vi "Calibrations.vi"() -> ()   [LabVIEW 2014]
panel:
  in  "Calibrations File Location":path=path "C:/ni-rt/startup/Calibrations.txt"
  in  "Gyro gain":dbl=0.007
  in  "Rear Right Encoder Correction Factor":dbl=1.17
  in  "Rear Left Encoder Correction Factor":dbl=5.99
  in  "Front Left Encoder Correction Factor":dbl=5.09
  in  "Front Right Encoder Correction Factor":dbl=1.3
  in  "Lift Encoder Calibration":dbl=1.0
  in  "Drive Encoder Calibration":dbl=1.0
  in  "Rear Left Encoder Max Voltage":dbl=4.94
  in  "Rear Left Encoder Min Voltage":dbl=0.01
  in  "Rear Right Encoder Max Voltage":dbl=4.94
  in  "Rear Right Encoder Min Voltage":dbl=0.01
  in  "Front Left Encoder Max Voltage":dbl=4.94
  in  "Front Left Encoder Min Voltage":dbl=0.01
  in  "Front Right Encoder Max Voltage":dbl=4.94
  in  "Front Right Encoder Min Voltage":dbl=0.015
  # "in/tick"
  # "Volts"
  # "in/tick"
  # "Volts"
  # "V/(deg*sec)"
  # "rad"
  # "Volts"
  # "Volts"
  # "rad"
  # "Volts"
  # "Volts"
  # "rad"
  # "Volts"
  # "Volts"
  # "rad"
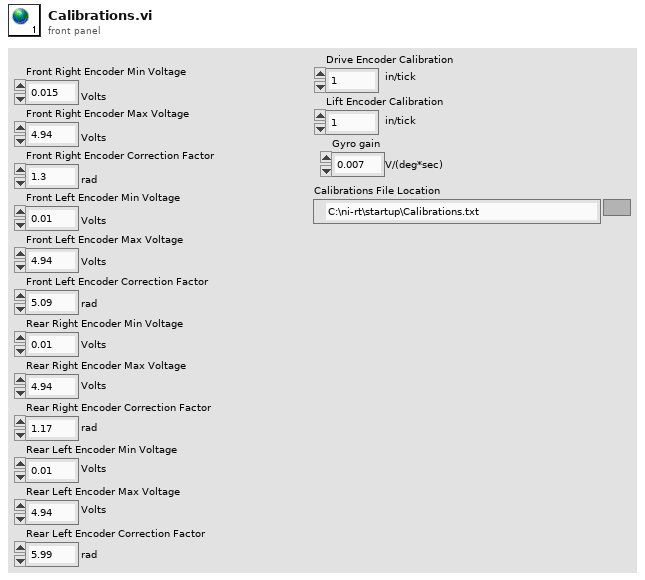
[diagram p1: front panel]
diagram:
